vi "2022 Auto Simple.vi"   [LabVIEW 2020]
uses:
  <vilib>/Rock Robotics/WPI/ThirdParty/Phoenix-LabVIEW/Motor Controller/Controls/CTRE_Phoenix_MotorControl_ControlMode.ctl
  <vilib>/Rock Robotics/WPI/Utilities/WPI_GetSetVariantRefNum.vi
types:
  T1 = typedef "CTRE_Phoenix_MotorControl_ControlMode.ctl" = u16
  T2 = typedef "WPI_RobotDriveDevRef.ctl" = cluster{"DevStatus":errorcluster, "Motors[]":T3[], "Square Inputs":bool, "Max Output":dbl}
  T3 = typedef "WPI_MotorControlDeviceRef.ctl" = cluster{"DeviceStatus":errorcluster, "Type":T4, "PWM":cluster{"PWM Channel":T5, "DeadBand":T6}, "CAN":cluster{"Device Number":u8, "SetOutput VI Ref":variant, "GetOutput VI Ref":variant, "Enable VI Ref":variant, "Disable VI Ref":variant, "Data":variant}, "Invert":bool, "DIO PWM":cluster{"PWM \"Enable\" Channel":T5, "DIOChannel":T7, "PWM Rate":dbl}}
  T4 = typedef "WPI_MotorControlType.ctl" = enum16{"PWM", "CAN", "DIO PWM"}
  T5 = typedef "FPGA_DIOPWMChannel.ctl" = enum8{"PWM 0", "PWM 1", "PWM 2", "PWM 3", "PWM 4", "PWM 5", "PWM 6", "PWM 7", "PWM 8", "PWM 9", "PWM MXP 0", "PWM MXP 1", "PWM MXP 2", "PWM MXP 3", "PWM MXP 4", "PWM MXP 5", "PWM MXP 6", "PWM MXP 7", "PWM MXP 8", "PWM MXP 9", "Invalid"}
  T6 = typedef "WPI_PWMDeadband.ctl" = cluster{"Name":string, "maxPositivePwm":i32, "minPositivePwm":i32, "centerPwm":i32, "maxNegativePwm":i32, "minNegativePwm":i32, "angularRange":u16}
  T7 = typedef "FPGA_DIOChannel.ctl" = enum8{"DIO 0", "DIO 1", "DIO 2", "DIO 3", "DIO 4", "DIO 5", "DIO 6", "DIO 7", "DIO 8", "DIO 9", "DIO MXP 0", "DIO MXP 1", "DIO MXP 2", "DIO MXP 3", "DIO MXP 4", "DIO MXP 5", "DIO MXP 6", "DIO MXP 7", "DIO MXP 8", "DIO MXP 9", "DIO MXP 10", "DIO MXP 11", "DIO MXP 12", "DIO MXP 13", "DIO MXP 14", "DIO MXP 15", "SPI Port CS1", "SPI Port CS2", "SPI Port CS3", "SPI Port MISO", "SPI Port MOSI", "Invalid"}
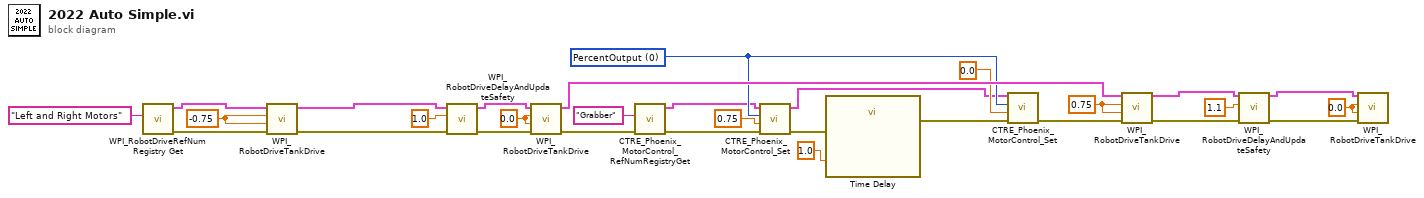
[diagram p0: block diagram]
diagram:
  w29 = 0.0 ("Output")
  w22 = 0.75 ("Left axis value")
  w9 = 0.0 ("Left axis value")
  w3 = -0.75 ("Left axis value")
  w20 = T1 0 items=["PercentOutput"=0, "Position"=1, "Velocity"=2, "Current"=3, "Follower"=5, "MotionProfile"=6, "MotionMagic"=7, "MotionProfileArc"=10, "Disabled"=15] ("Control Mode")
  n1 = call <vilib>:"WPI_RobotDriveRefNum Registry Get.vi"("refnum name"="Left and Right Motors") -> ("error out"=w4:errorcluster, "RobotDriveDevRef"=w2:T2)  [unwired: 1 in, 8 out]
  n2 = call <vilib>:"WPI_RobotDriveTankDrive.vi"("error in (no error)"=w4, "Right axis value"=w3, "Left axis value"=w3, "RobotDriveDevRef"=w2) -> ("error out"=w7:errorcluster, "RobotDriveDevRef"=w5:T2)  [unwired: 5 in, 1 out]
  n3 = call <vilib>:"WPI_RobotDriveDelayAndUpdateSafety.vi"("error in (no error)"=w7, "Delay (s)"=1.0, "RobotDriveDevRef"=w5) -> ("error out"=w10:errorcluster, "RobotDriveDevRef 2"=w8:T2)  [unwired: 7 in]
  n4 = call <vilib>:"WPI_RobotDriveTankDrive.vi"("error in (no error)"=w10, "Right axis value"=w9, "Left axis value"=w9, "RobotDriveDevRef"=w8) -> ("error out"=w15:errorcluster, "RobotDriveDevRef"=w23:T2)  [unwired: 5 in, 1 out]
  n5 = call <vilib>:"CTRE_Phoenix_MotorControl_RefNumRegistryGet.vi"("error in (no error)"=w15, "refnum name"="Grabber") -> ("error out"=w14:errorcluster, "PhoenixMotorControlDevRef"=w12:T3)  [unwired: 8 in]
  n6 = call <vilib>:"CTRE_Phoenix_MotorControl_Set.vi"("error in (no error)"=w14, "Output"=0.75, "Control Mode"=w20, "PhoenixMotorControlDevRef"=w12) -> ("error out"=w17:errorcluster, "PhoenixMotorControlDevRef"=w18:T3)  [unwired: 6 in]
  n7 = call "Time Delay"("error in (no error)"=w17, "Delay Time (s)"=1.0) -> ("error out"=w21:errorcluster)  [unwired: 9 in]
  n8 = call <vilib>:"CTRE_Phoenix_MotorControl_Set.vi"("error in (no error)"=w21, "Output"=0.0, "Control Mode"=w20, "PhoenixMotorControlDevRef"=w18) -> ("error out"=w24:errorcluster)  [unwired: 6 in, 1 out]
  n9 = call <vilib>:"WPI_RobotDriveTankDrive.vi"("error in (no error)"=w24, "Right axis value"=w22, "Left axis value"=w22, "RobotDriveDevRef"=w23) -> ("error out"=w25:errorcluster, "RobotDriveDevRef"=w26:T2)  [unwired: 5 in, 1 out]
  n10 = call <vilib>:"WPI_RobotDriveDelayAndUpdateSafety.vi"("error in (no error)"=w25, "Delay (s)"=1.1, "RobotDriveDevRef"=w26) -> ("error out"=w30:errorcluster, "RobotDriveDevRef 2"=w28:T2)  [unwired: 7 in]
  n11 = call <vilib>:"WPI_RobotDriveTankDrive.vi"("error in (no error)"=w30, "Right axis value"=w29, "Left axis value"=w29, "RobotDriveDevRef"=w28) -> ()  [unwired: 5 in, 3 out]
